vi "SetCompliance.vi"(3 "Current":sgl=0.011, 4 "Voltage":sgl=21.0, 5 "Device":u8=1, 6 "Serial port":refnum<visa-resource-name>) -> (1 "Device out":u8=1, 2 "Serial port out":refnum<visa-resource-name>)   [LabVIEW 2021]
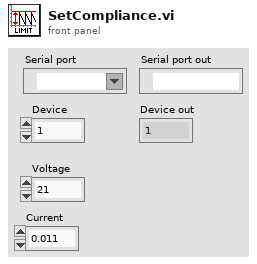
[diagram p1: front panel]
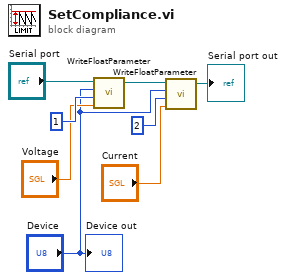
[diagram p0: block diagram]
diagram:
  n1 = call "WriteFloatParameter.vi"("Value"="Voltage", "Address"=u32 1, "Device"="Device", "Serial port"="Serial port") -> ("Serial port out"=w8:refnum<visa-resource-name>)  [unwired: 2 in]
  n2 = call "WriteFloatParameter.vi"("Value"="Current", "Address"=u32 2, "Device"="Device", "Serial port"=w8) -> ("Serial port out"=→"Serial port out":refnum<visa-resource-name>)  [unwired: 2 in]
  "Device out" <- "Device"
